vi "OCULOGRAMA_LED.vi"() -> ()   [LabVIEW 2016]
uses:
  <vilib>/LabVIEW Interface for Arduino/LabVIEW Interface for Arduino.lvlib
  <vilib>/LabVIEW Interface for Arduino/Type Defs/Board Type.ctl
panel:
  out "ABAJO":bool
  out "ARRIBA":bool
  out "DERECHA":bool
  out "IZQUIERDA":bool
  in  "Arriba":dbl
  in  "Abajo":dbl
  in  "DERECHA":dbl
  in  "IZQUIERDA":dbl
  out "Vertical":dbl(graph) caption="Waveform Chart"
  in  "stop":bool
  out "Horizontal":dbl(graph) caption="Waveform Chart"
  # "Condicionales"
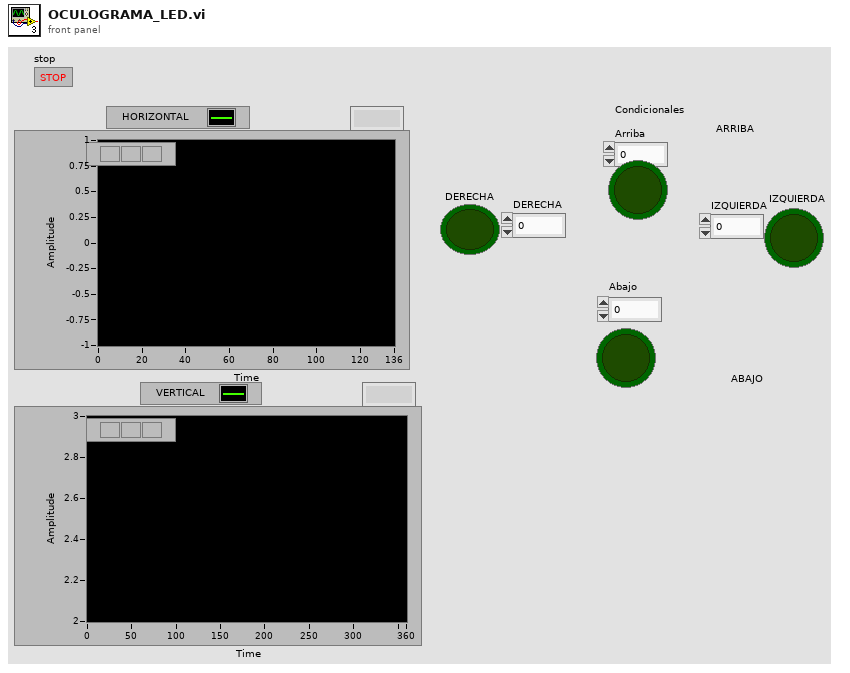
[diagram p1: front panel]
types:
  T1 = typedef "LabVIEW Interface for Arduino.lvlib/Board Type.ctl" = enum16{"Uno", "Dimuelanove w/Atmega 328", "Mega 2560"}
  T2 = typedef "LabVIEW Interface for Arduino.lvlib/Arduino Resource.ctl" = cluster{"VISA resource":refnum<visa-resource-name>, "Board Type":T1, "Connection Type":enum8{"USB / Serial"}, "Bytes Per Packet (15)":u8}
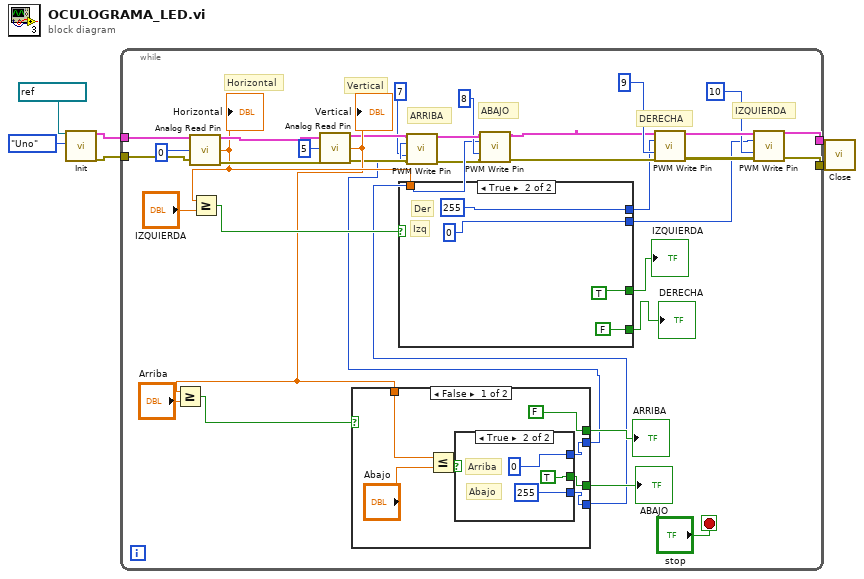
[diagram p0: block diagram]
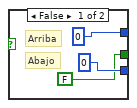
[diagram p2: hidden frame]
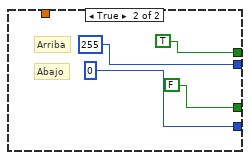
[diagram p3: hidden frame]
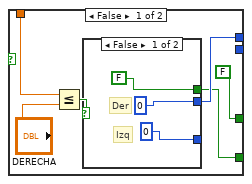
[diagram p4: hidden frame]
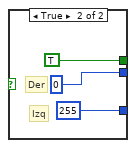
[diagram p5: hidden frame]
diagram:
  n1 = call <vilib>:"Init.vi"("VISA resource"=refnum<visa-resource-name> "COM11", "Board Type (Uno)"=Board_Type."Uno") -> ("Arduino Resource"=w6:T2, "error out"=w5:errorcluster)  [unwired: 16 in]
  n2 = while {
    tunnel: w6 -> [w40]
    tunnel: w5 -> [w39]
    tunnel: [w11] -> w2
    tunnel: [w10] -> w1
    stop <- "stop" stop-if-true
    # "ABAJO"
    # "ARRIBA"
    # "IZQUIERDA"
    # "DERECHA"
    # "Vertical"
    # "Horizontal"
    n3 = call <vilib>:"Analog Read Pin.vi"("Arduino Resource"=w40, "Analog Input Pin (0)"=u8 0, "error in"=w39) -> ("Arduino Resource"=w37:T2, "Voltage"=w31:dbl, "error out"=w36:errorcluster)  [unwired: 10 in]
    "Horizontal" <- w31
    n4 = Greater Or Equal?(x=w31, y="IZQUIERDA") -> (x >= y?=w32:bool)
    n5 = call <vilib>:"Analog Read Pin.vi"("Arduino Resource"=w37, "Analog Input Pin (0)"=u8 5, "error in"=w36) -> ("Arduino Resource"=w23:T2, "Voltage"=w28:dbl, "error out"=w22:errorcluster)  [unwired: 10 in]
    "Vertical" <- w28
    n6 = Greater Or Equal?(x=w28, y="Arriba") -> (x >= y?=w29:bool)
    n7 = case shown="False" w29 {
      tunnel: [w44 255] -> w21
      tunnel: [w43 0] -> w17
      tunnel: w28 -> [w45 _]
      tunnel: [FALSE TRUE] -> w25
      tunnel: [w41 FALSE] -> w24
      frame False {
        n8 = Less Or Equal?(x=w45, y="Abajo") -> (x <= y?=w46:bool)
        n9 = case shown="True" w46 {
          tunnel: [0 0] -> w44
          tunnel: [0 255] -> w43
          tunnel: [FALSE TRUE] -> w41
          frame False {
            # "Abajo"
            # "Arriba"
          }
          frame True {
            # "Abajo"
            # "Arriba"
          }
        }
      }
      frame True {
        # "Abajo"
        # "Arriba"
      }
    }
    "ARRIBA" <- w25
    "ABAJO" <- w24
    n10 = case shown="True" w32 {
      tunnel: [w60 255] -> w13
      tunnel: w31 -> [w61 _]
      tunnel: [FALSE TRUE] -> w27
      tunnel: [w58 FALSE] -> w26
      tunnel: [_ 0] -> w7
      frame False {
        n11 = Less Or Equal?(x=w61, y="DERECHA") -> (x <= y?=w62:bool)
        n12 = case shown="False" w62 {
          tunnel: [0 0] -> w60
          tunnel: [0 255] -> _
          tunnel: [FALSE TRUE] -> w58
          frame False {
            # "Izq"
            # "Der"
          }
          frame True {
            # "Izq"
            # "Der"
          }
        }
      }
      frame True {
        # "Izq"
        # "Der"
      }
    }
    "IZQUIERDA" <- w27
    "DERECHA" <- w26
    n13 = call <vilib>:"PWM Write Pin.vi"("Arduino Resource"=w23, "Duty Cycle (0 - 255)"=w21, "PWM Pin (3)"=u8 7 ("Digital I/O Pin (0)"), "error in"=w22) -> ("Arduino Resource"=w19:T2, "error out"=w16:errorcluster)  [unwired: 10 in]
    n14 = call <vilib>:"PWM Write Pin.vi"("Arduino Resource"=w19, "Duty Cycle (0 - 255)"=w17, "PWM Pin (3)"=u8 8 ("Digital I/O Pin (0)"), "error in"=w16) -> ("Arduino Resource"=w12:T2, "error out"=w15:errorcluster)  [unwired: 10 in]
    n15 = call <vilib>:"PWM Write Pin.vi"("Arduino Resource"=w12, "Duty Cycle (0 - 255)"=w13, "PWM Pin (3)"=u8 9 ("Digital I/O Pin (0)"), "error in"=w15) -> ("error out"=w9:errorcluster)  [unwired: 10 in, 1 out]
    n16 = call <vilib>:"PWM Write Pin.vi"("Arduino Resource"=w12, "Duty Cycle (0 - 255)"=w7, "PWM Pin (3)"=u8 10 ("Digital I/O Pin (0)"), "error in"=w9) -> ("Arduino Resource"=w11:T2, "error out"=w10:errorcluster)  [unwired: 10 in]
  }
  n17 = call <vilib>:"Close.vi"("Arduino Resource"=w2, "error in"=w1) -> ()  [unwired: 13 in, 1 out]
